vi "Get-TestCases.vi"(8 "error in (no error)":errorcluster) -> (0 "error out":errorcluster, 3 "value":T1)   [LabVIEW 2018, in "Launcher Main Module.lvlib"]
uses:
  Launcher Main Module.lvlib
  Module_Controls/Google_Sheet_Test_Case.ctl
  <vilib>/httpClient/LabVIEWHTTPClient.lvlib
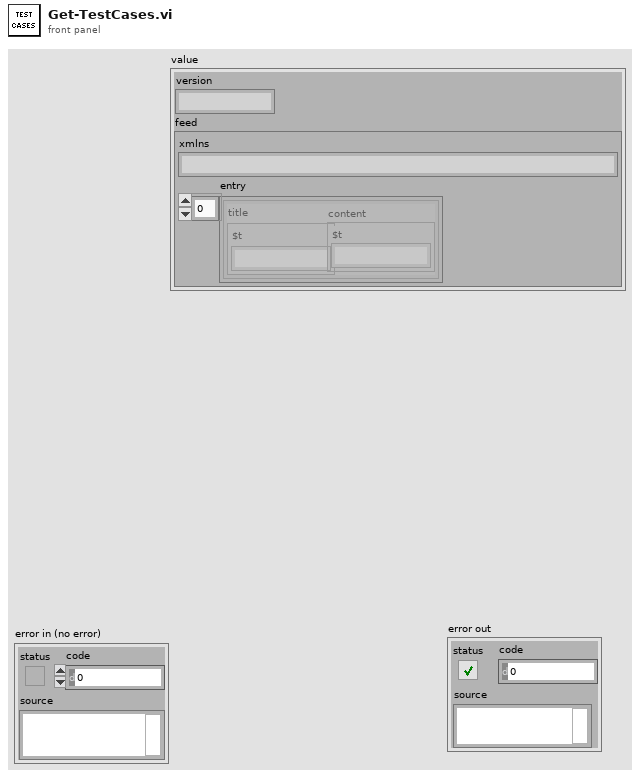
[diagram p1: front panel]
types:
  T1 = typedef "Launcher Main Module.lvlib/Google_Sheet_Test_Case.ctl" = cluster{"version":string, "feed":cluster{"xmlns":string, "entry":cluster{"title":cluster{"$t":string}, "content":cluster{"$t":string}}[]}}
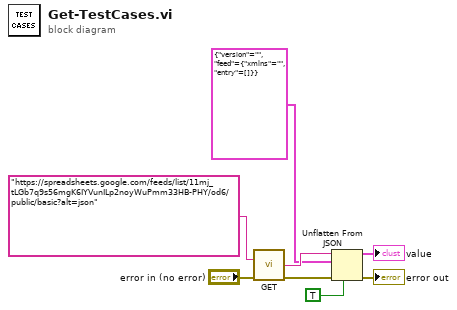
[diagram p0: block diagram]
diagram:
  n1 = call <vilib>:"GET.vi"("url"="https://spreadsheets.google.com/feeds/list/11mj_tLGb7q9s56mgK6IYVunILp2noyWuPmm33HB-PHY/od6/public/basic?alt=json", "error in (no error)"="error in (no error)") -> ("body"=w7:string, "error out"=w4:errorcluster)  [unwired: 10 in, 2 out]
  n2 = Unflatten From JSON(JSON string=w7, type and defaults=T1 {"version"="", "feed"={"xmlns"="", "entry"=[]}} ("value"), default null elements? (F)=TRUE, error in (no error)=w4) -> (value=→"value":T1, error out=→"error out":errorcluster)  [unwired: 3 in]
